vi "Create GUID.vi"(8 "error in (no error)":errorcluster) -> (0 "error out":errorcluster, 3 "GUID":string)   [LabVIEW 2011]
doc: "GUID stands for <B>G</B>lobally <B>U</B>nique <B>ID</B>entifier, a 128-bit integer used as unique identifier.\n\nThis VI makes a call to ole32.dll to create an absolutely unique number that you can use as a persistent identifier in a distributed environment.To a very high degree of certainty, this function returns a unique value: no other invocation, on the same or any other system (networked or not), should return the same value.\n\n<B>GUID Cluster</B> returns the GUID in a cluster that follows the GUID format.\n\n<B>GUID String</B> has the GUID as a string of characters.\n\n<B>GUID OLE String</B> has a format like that of the following sample:\n\n{c200e360-38c5-11ce-ae62-08002b2b79ef} \n \nwhere the successive fields break the GUID into the form:\n\nDWORD-WORD-WORD-WORD-WORD-DWORD\n\ncovering the 128-bit GUID. The string includes the enclosing braces, which are an OLE convention.\n\nEnrique Vargas\nvargas@jyestudio.com"
panel:
  out "GUID String":string
  out "GUID OLE String":string
  out "GUID Cluster":T1 {"Data4" format="%.0x"; "Data3" format="%.0x"; "Data2" format="%.0x"; "Data1" format="%.0x"}
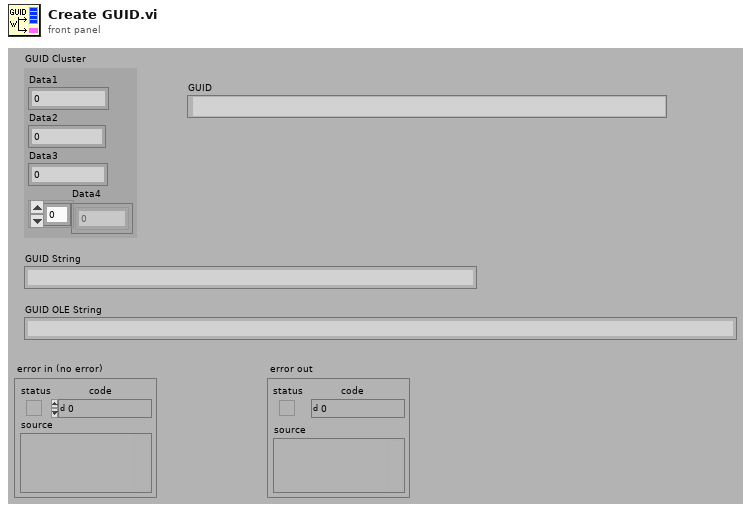
[diagram p1: front panel]
types:
  T1 = cluster{"Data1":u32, "Data2":u16, "Data3":u16, "Data4":u8[]}
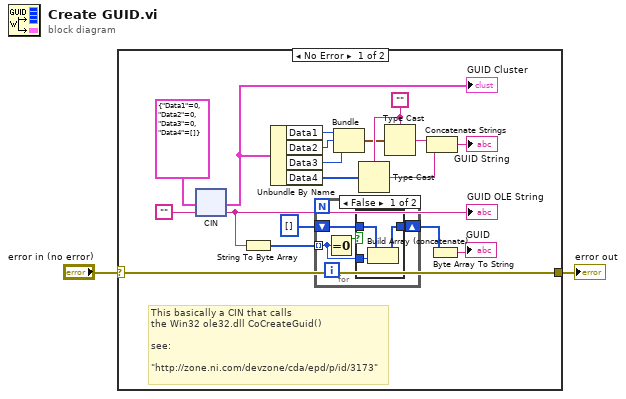
[diagram p0: block diagram]
diagram:
  n1 = case shown="No Error" "error in (no error)" {
    selector: "error in (no error)" -> [w8 w29]
    tunnel: [w8 w29] -> w1
    frame No Error {
      w14 = ""
      # "This basically a CIN that calls\nthe Win32 ole32.dll CoCreateGuid()\n\nsee:\n\n\"http://zone.ni.com/devzone/cda/epd/p/id/3173\""
      n2 = cin(T1 {"Data1"=0, "Data2"=0, "Data3"=0, "Data4"=[]} ("GUID"), "") -> (w10:T1, w7:string)
      "GUID Cluster" <- w10
      "GUID OLE String" <- w7
      n3 = String To Byte Array(string=w7) -> (unsigned byte array=w6:u8[])
      n4 = Unbundle By Name(w10) -> ("Data1"=w18:u32, "Data2"=w17:u16, "Data3"=w16:u16, "Data4"=w12:u8[])
      n5 = for {
        tunnel: w6 -> [w22] mode=indexing
        shift-right: [w23] -> w4
        shift-left: u8[] [] ("unsigned byte array") -> [w24]
        n6 = Equal To 0?(x=w22) -> (x = 0?=w21:bool)
        n7 = case shown="False" w21 {
          tunnel: w24 -> [w27 w28]
          tunnel: [w26 w28] -> w23
          tunnel: w22 -> [w25 _]
          frame False {
            n8 = Build Array (concatenate)(w27, w25) -> (w26:u8[])
          }
          frame True {
          }
        }
      }
      n9 = Bundle("Data1"=w18, "Data2"=w17, "Data3"=w16) -> (w11:cluster{"Data1":u32, "Data2":u16, "Data3":u16})  [unwired: 1 in]
      n10 = Type Cast(type=w14, x=w12) -> (*(type *) &x=w13:string)
      n11 = Type Cast(type=w14, x=w11) -> (*(type *) &x=w15:string)
      n12 = Concatenate Strings(w15, w13) -> (→"GUID String":string)
      n13 = Byte Array To String(unsigned byte array=w4) -> (string=→"GUID":string)
    }
    frame Error {
    }
  }
  "error out" <- w1
